vi "Poll Sensor Group 0.vi"(8 "error in":errorcluster, 11 "UART port in":T6) -> (0 "error out":errorcluster, 1 "Timed Out?":bool, 2 "Sensor Group 0":T1={"Bumps + Wheel Drops"={"Wheeldrop Caster"=FALSE, "Wheeldrop Left"=FALSE, "Wheeldrop Right"=FALSE, "Bump Left"=FALSE, "Bump Right"=FALSE}, "Wall"=FALSE, "Cliff Left"=FALSE, "Cliff Front Left"=FALSE, "Cliff Front Right"=FALSE, "Cliff Right"=FALSE, "Virtual Wall"=FALSE, "Low-Side Driver + Wheel Overcurrent"={"Low-Side Driver 0"=FALSE, "Low-Side Driver 1"=FALSE, "Low-Side Driver 2"=FALSE, "Left Wheel"=FALSE, "Right Wheel"=FALSE}, "Infrared"=255, "Buttons"={"Advance"=FALSE, "Play"=FALSE}, "Distance (mm)"=0, "Angle (deg)"=0, "Charging State"=enum."Not Charging", "Voltage (mV)"=0, "Current (mA)"=0, "Battery Temperature (deg C)"=0, "Battery Charge (mAh)"=0, "Battery Capacity (mAh)"=0} {"Infrared" format="%02x"}, 3 "UART port out":T6)   [LabVIEW 2013]
doc: "Poll the iRobot for Sensor Group 0; blocks until response is received, or the operation has timed out.\n\nThis VI both writes to AND reads from the serial port.\n<b>NOTE</b>: This should not be used in a loop if other serial reading or writing VIs are called in parallel loops."
uses:
  Advanced/UART/iRobot UART Port Type.ctl
  Sensor Group 0.ctl
  Bumps + Wheel Drops.ctl
  Low-Side Driver + Wheel Overcurrent.ctl
  Buttons.ctl
  Charging State.ctl
  Sensor ID.ctl
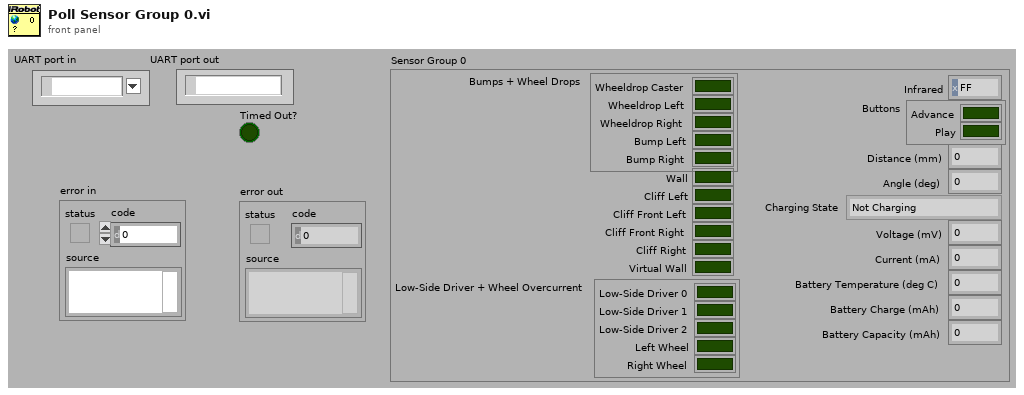
[diagram p1: front panel]
types:
  T1 = typedef "Sensor Group 0.ctl" = cluster{"Bumps + Wheel Drops":T2, "Wall":bool, "Cliff Left":bool, "Cliff Front Left":bool, "Cliff Front Right":bool, "Cliff Right":bool, "Virtual Wall":bool, "Low-Side Driver + Wheel Overcurrent":T3, "Infrared":u8, "Buttons":T4, "Distance (mm)":i32, "Angle (deg)":i32, "Charging State":T5, "Voltage (mV)":u16, "Current (mA)":i16, "Battery Temperature (deg C)":i8, "Battery Charge (mAh)":u16, "Battery Capacity (mAh)":u16}
  T2 = typedef "Bumps + Wheel Drops.ctl" = cluster{"Wheeldrop Caster":bool, "Wheeldrop Left":bool, "Wheeldrop Right":bool, "Bump Left":bool, "Bump Right":bool}
  T3 = typedef "Low-Side Driver + Wheel Overcurrent.ctl" = cluster{"Low-Side Driver 0":bool, "Low-Side Driver 1":bool, "Low-Side Driver 2":bool, "Left Wheel":bool, "Right Wheel":bool}
  T4 = typedef "Buttons.ctl" = cluster{"Advance":bool, "Play":bool}
  T5 = typedef "Charging State.ctl" = enum16{"Not Charging", "Reconditioning Charging", "Full Charging", "Trickle Charging", "Waiting", "Charging Fault Condition"}
  T6 = typedef "iRobot UART Port Type.ctl" = refnum<visa-resource-name>
  T7 = typedef "Sensor ID.ctl" = enum8{"Sensor Group 0", "Sensor Group 1", "Sensor Group 2", "Sensor Group 3", "Sensor Group 4", "Sensor Group 5", "Sensor Group 6", "Bump + Wheel Drop", "Wall", "Cliff Left", "Cliff Front Left", "Cliff Front Right", "Cliff Right", "Virtual Wall", "Low Side Driver + Wheel Overcurrent", "Unused 0", "Unused 1", "Infrared", "Buttons", "Distance", "Angle", "Charging State", "Voltage", "Current", "Battery Temperature", "Battery Charge", "Battery Capacity", "Wall Signal", "Cliff Left Signal", "Cliff Front Left Signal", "Cliff Front Right Signal", "Cliff Right Signal", "Cargo Bay Digital Inputs", "Cargo Bay Analog Signal", "Charging Sources Available", "OI Mode", "Song Number", "Song Playing", "Number of Stream Packets", "Requested Velocity", "Requested Radius", "Requested Right Velocity", "Requested Left Velocity"}
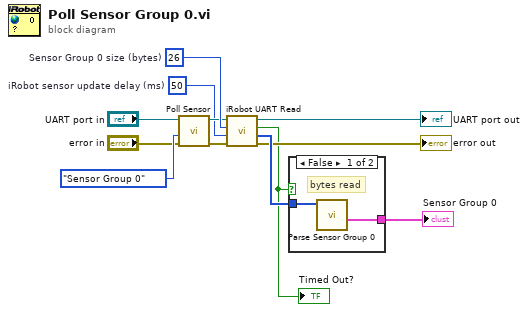
[diagram p0: block diagram]
diagram:
  w3 = 50  # iRobot sensor update delay (ms)
  w11 = 26  # Sensor Group 0 size (bytes)
  n1 = call "Poll Sensor.vi"("error in"="error in", "Sensor ID"=Sensor_ID."Sensor Group 0", "UART port in"="UART port in") -> ("error out"=w6:errorcluster, "UART port out"=w9:T6)  [unwired: 7 in]
  n2 = call "iRobot UART Read.vi"("error in"=w6, "timeout (ms)"=w3, "Number of Bytes"=w11, "UART port in"=w9) -> ("error out"=→"error out":errorcluster, "UART Stream"=w10:u8[], "Timed Out?"=w2:bool, "UART port out"=→"UART port out":T6)  [unwired: 4 in]
  "Timed Out?" <- w2
  n3 = case shown="False" w2 {
    tunnel: w10 -> [w14 _]
    tunnel: [w13 _] -> w1
    frame False {
      # "bytes read"
      n4 = call "Parse Sensor Group 0.vi"("stream in"=w14) -> ("Sensor Group 0"=w13:T1)  [unwired: 9 in, 1 out]
    }
    frame True {
      # "timeout"
    }
  }
  "Sensor Group 0" <- w1
